vi "ATF-Pump-Drive A_D-DP FGV.vi"(7 "Write/Read":T1=enum."Read", 8 "error in (no error)":errorcluster, 11 "Drive A_D":waveform(dbl)[](array[waveform])) -> (0 "error Out":errorcluster, 3 "Drive A_D data":waveform(dbl)[](array[waveform]))   [LabVIEW 2022 SP3]
uses:
  RT Controls/ATF-Pump-FGV Read write.ctl
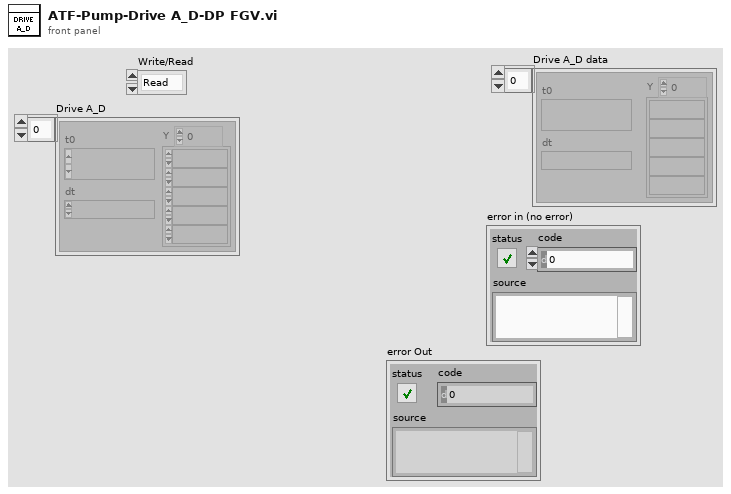
[diagram p1: front panel]
types:
  T1 = typedef "ATF-Pump-FGV Read write.ctl" = enum16{"Write", "Read"}
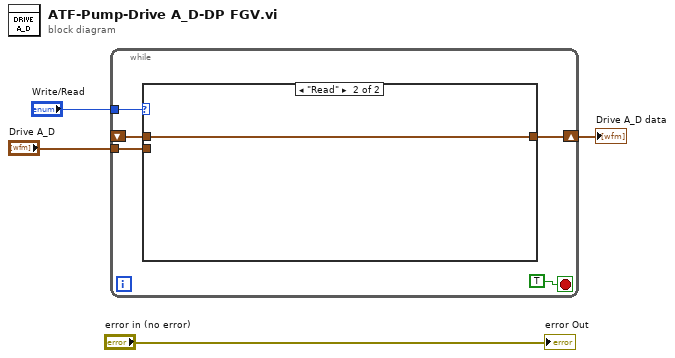
[diagram p0: block diagram]
diagram:
  n1 = while {
    tunnel: "Write/Read" -> [w8]
    shift-right: [w7] -> w3
    shift-left: _ -> [w6]
    tunnel: "Drive A_D" -> [w5]
    stop <- TRUE stop-if-true
    n2 = case shown="\"Read\"" w8 {
      tunnel: [w10 w11] -> w7
      tunnel: w6 -> [_ w11]
      tunnel: w5 -> [w10 _]
      frame "Write" {
      }
      frame "Read" {
      }
    }
  }
  "Drive A_D data" <- w3
  "error Out" <- "error in (no error)"
